vi "update.vi"(8 "error in (no error)":errorcluster, 10 "ExperimentVariables (in)":refnum<class "ExperimentVariables.lvclass">, 11 "Analog_Output in":refnum<class "Analog_Output.lvclass">) -> (0 "error out":errorcluster, 2 "ExperimentVariables":refnum<class "ExperimentVariables.lvclass">, 3 "Analog_Output out":refnum<class "Analog_Output.lvclass">)   [LabVIEW 2013, in "Analog_Output.lvclass"]
uses:
  Analog_Output.lvclass
  <vilib>/DAQmx/write.llb/DAQmx Write (Analog 1D Wfm NChan NSamp).vi
  ExperimentVariables/ExperimentVariables.lvclass
  <vilib>/DAQmx/configure/timing.llb/DAQmx Timing (Sample Clock).vi
  <vilib>/gmath/NI_Gmath.lvlib
panel:
  out "Waveform Graph":waveform(dbl)[](graph)
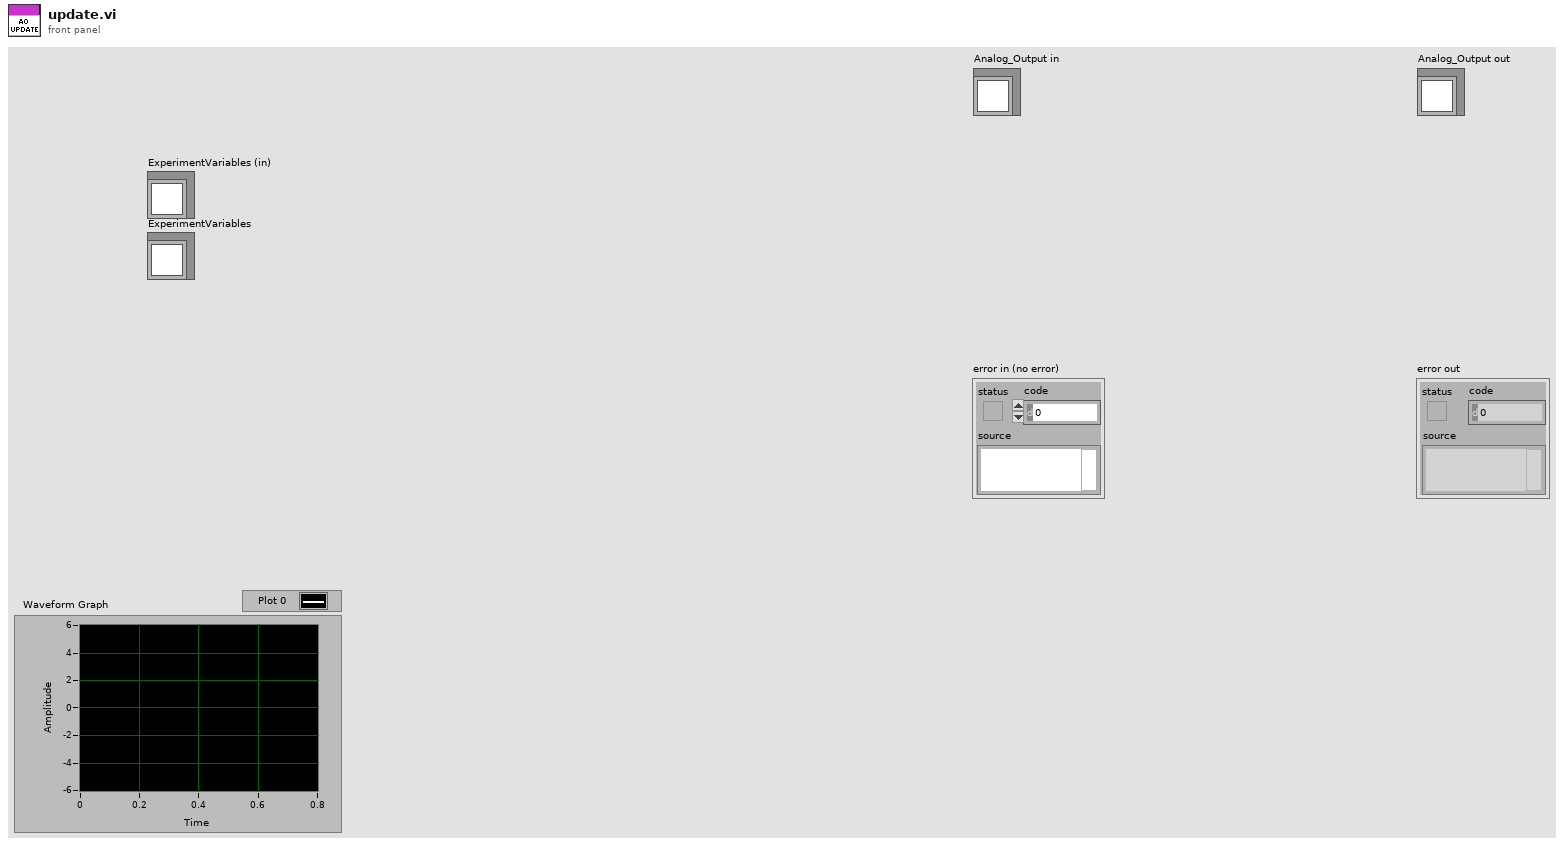
[diagram p1: front panel]
types:
  T1 = cluster{"Wait for start trigger?":bool, "source":tag, "edge":i32}
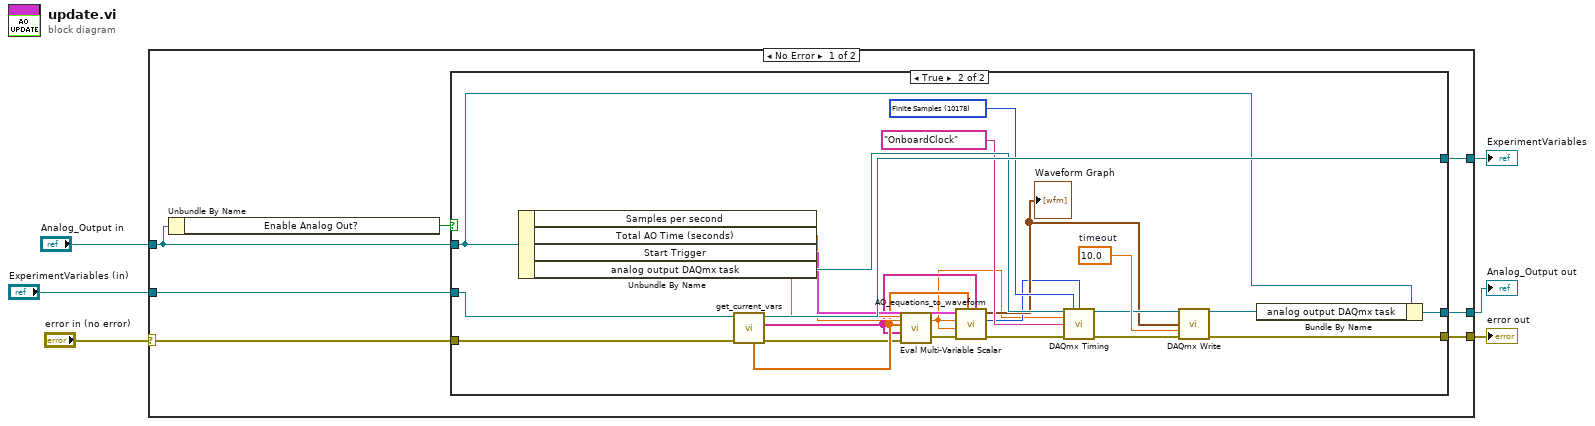
[diagram p0: block diagram]
diagram:
  n1 = case shown="No Error" "error in (no error)" {
    selector: "error in (no error)" -> [w13 w43]
    tunnel: [w12 w43] -> w5
    tunnel: [w8 w42] -> w3
    tunnel: "Analog_Output in" -> [w9 w42]
    tunnel: "ExperimentVariables (in)" -> [w11 w41]
    tunnel: [w10 w41] -> w1
    frame No Error {
      n2 = Unbundle By Name(w9) -> ("Enable Analog Out?"=w7:bool)
      n3 = case shown="True" w7 {
        tunnel: w13 -> [w16 w39]
        tunnel: [w16 w36] -> w12
        tunnel: w11 -> [w15 w38]
        tunnel: [w15 w37] -> w10
        tunnel: w9 -> [w14 w35]
        tunnel: [w14 w34] -> w8
        frame False {
        }
        frame True {
          w32 = 10178 items=["Finite Samples"=10178, "Continuous Samples"=10123, "Hardware Timed Single Point"=12522] ("sample mode")
          w40 = 10.0  # timeout
          n4 = Unbundle By Name(w35) -> ("Samples per second"=w22:dbl, "Total AO Time (seconds)"=w27:dbl, "Start Trigger"=w28:T1, "analog output DAQmx task"=w31:refnum<k21>)
          n5 = call-dynamic "get_current_vars.vi"("error in (no error)"=w39, "ExperimentVariables in"=w38) -> ("error out"=w18:errorcluster, "variables and parameter names"=w20:string[], "ExperimentVariables out"=w37:refnum<class "ExperimentVariables.lvclass">, "current variable and parameter values"=w21:dbl[])  [unwired: 4 in, 2 out]
          n6 = call <vilib>:"Eval Multi-Variable Scalar.vi"("error in (no error)"=w18, "Variables"=w20, "X Values"=w21, "formula"=w22) -> ("error out"=w17:errorcluster, "y value"=w19:dbl)
          n7 = call "AO_equations_to_waveform.vi"("variable/parameter names"=w20, "minimum/current values"=w21, "error in (no error)"=w17, "Samples per second"=w19, "Total AO Time"=w27, "Analog Output Equations for each Channel"=w28) -> ("error out"=w24:errorcluster, "Total # Samples"=w25:i32, "Waveform Graph"=w26:waveform(dbl)[])  [unwired: 3 in]
          "Waveform Graph" <- w26
          n8 = call-poly <vilib>:"DAQmx Timing.vi"("task/channels in"=w31, "sample mode"=w32, "samples per channel"=w25, "rate"=w19, "source"=tag "OnboardClock", "error in"=w24) -> ("task out"=w30:refnum<k21>, "error out"=w23:errorcluster)  [unwired: 8 in]
          n9 = call-poly <vilib>:"DAQmx Write.vi"("task/channels in"=w30, "data"=w26, "timeout"=w40, "error in"=w23) -> ("task out"=w33:refnum<k21>, "error out"=w36:errorcluster)  [unwired: 9 in, 1 out]
          n10 = Bundle By Name(cluster=w35, "analog output DAQmx task"=w33) -> (w34:refnum<class "Analog_Output.lvclass">)
        }
      }
    }
    frame Error {
    }
  }
  "error out" <- w5
  "Analog_Output out" <- w3
  "ExperimentVariables" <- w1
